vi "Sensors_Scale.vi"() -> ()   [LabVIEW 2017]
uses:
  <vilib>/DAQmx/read.llb/DAQmx Read (Analog 1D Wfm NChan NSamp).vi
  <vilib>/DAQmx/miscellaneous.llb/DAQmx Fill In Error Info.vi
panel:
  out "weight (g)":dbl format="%#_13g"
  out "?":cluster{timestamp[], dbl[]}(graph)={[timestamp(3602780680.000294 s since 1904-01-01), timestamp(3602780680.1853123 s since 1904-01-01), timestamp(3602780680.372331 s since 1904-01-01), timestamp(3602780680.5593495 s since 1904-01-01), timestamp(3602780680.747369 s since 1904-01-01), timestamp(3602780680.9313874 s since 1904-01-01), timestamp(3602780681.120406 s since 1904-01-01), timestamp(3602780681.309425 s since 1904-01-01), timestamp(3602780681.4954433 s since 1904-01-01), timestamp(3602780681.6844625 s since 1904-01-01), timestamp(3602780681.871481 s since 1904-01-01), timestamp(3602780682.0585 s since 1904-01-01), timestamp(3602780682.2445183 s since 1904-01-01), timestamp(3602780682.4305367 s since 1904-01-01), timestamp(3602780682.6185555 s since 1904-01-01), timestamp(3602780682.8075743 s since 1904-01-01), timestamp(3602780682.9955935 s since 1904-01-01), timestamp(3602780683.183612 s since 1904-01-01), timestamp(3602780683.371631 s since 1904-01-01), timestamp(3602780683.56065 s since 1904-01-01), timestamp(3602780683.7476687 s since 1904-01-01), timestamp(3602780683.9326873 s since 1904-01-01), timestamp(3602780684.1167054 s since 1904-01-01), timestamp(3602780684.304724 s since 1904-01-01), timestamp(3602780684.492743 s since 1904-01-01), timestamp(3602780684.680762 s since 1904-01-01), timestamp(3602780684.8677807 s since 1904-01-01), timestamp(3602780685.0578 s since 1904-01-01), timestamp(3602780685.244818 s since 1904-01-01), timestamp(3602780685.432837 s since 1904-01-01)], [0.21837152908225832, 0.21742377911483501, 0.21031033814915645, 0.2086503005079301, 0.21884613322679414, 0.22074219760114033, 0.21125840768619142, 0.21932122763939432, 0.23473182361237477, 0.2444530148877071, 0.20770159564161617, 0.22524839457404866, 0.22667064865852637, 0.20628031893126675, 0.2335451032209548, 0.2169493088130814, 0.23188682444882147, 0.2193204281648633, 0.23781582193533168, 0.2190824597701706, 0.22382541061956118, 0.20746577490400142, 0.21813546462485434, 0.2209789641439528, 0.2205049837107893, 0.2292782030754168, 0.21410368192326956, 0.223114304440994, 0.2330717025481377, 0.23520626745287387]}
  in  "Clear Data":bool
  out "output cluster":T1={"Dynamic Data"=[{"t0"=timestamp(3602781702.123506 s since 1904-01-01), "dt"=0.001, "Y"=[-49.920074642439154, -49.92818457064587, -49.93629449885258, -49.93629449885258, -49.92818457064587, -49.91196471423243, -49.93629449885258, -49.944404427059304, -49.920074642439154, -49.920074642439154, -49.93629449885258, -49.93629449885258, -49.93629449885258, -49.920074642439154, -49.93629449885258, -49.93629449885258, -49.93629449885258, -49.92818457064587, -49.93629449885258, -49.92818457064587, -49.96062428347275, -49.92818457064587, -49.91196471423243, -49.93629449885258, -49.93629449885258, -49.92818457064587, -49.92818457064587, -49.920074642439154, -49.93629449885258, -49.93629449885258, -49.93629449885258, -49.920074642439154, -49.92818457064587, -49.952514355266025, -49.92818457064587, -49.92818457064587, -49.93629449885258, -49.92818457064587, -49.92818457064587, -49.93629449885258, -49.92818457064587, -49.93629449885258, -49.944404427059304, -49.93629449885258, -49.920074642439154, -49.92818457064587, -49.944404427059304, -49.93629449885258, -49.93629449885258, -49.92818457064587, -49.92818457064587, -49.93629449885258, -49.92818457064587, -49.920074642439154, -49.93629449885258, -49.93629449885258, -49.93629449885258, -49.920074642439154, -49.920074642439154, -49.93629449885258, -49.93629449885258, -49.920074642439154, -49.93629449885258, -49.93629449885258, -49.92818457064587, -49.92818457064587, -49.93629449885258, -49.92818457064587, -49.944404427059304, -49.93629449885258, -49.91196471423243, -49.92818457064587, -49.952514355266025, -49.952514355266025, -49.920074642439154, -49.92818457064587, -49.952514355266025, -49.92818457064587, -49.92818457064587, -49.92818457064587, -49.92818457064587, -49.93629449885258, -49.92818457064587, -49.91196471423243, -49.920074642439154, -49.92818457064587, -49.92818457064587, -49.920074642439154, -49.92818457064587, -49.944404427059304, -49.93629449885258, -49.91196471423243, -49.944404427059304, -49.93629449885258, -49.93629449885258, -49.920074642439154, -49.93629449885258, -49.944404427059304, -49.944404427059304, -49.92818457064587], "attributes"=variant("NI_ChannelName"=variant(string "CCP"), "NI_UnitDescription"=variant(string "psi"))}, {"t0"=timestamp(3602781702.12352 s since 1904-01-01), "dt"=0.001, "Y"=[-49.944404427059304, -49.920074642439154, -49.944404427059304, -49.92818457064587, -49.92818457064587, -49.96062428347275, -49.93629449885258, -49.90385478602571, -49.92818457064587, -49.96062428347275, -49.92818457064587, -49.91196471423243, -49.920074642439154, -49.93629449885258, -49.93629449885258, -49.92818457064587, -49.92818457064587, -49.93629449885258, -49.96062428347275, -49.93629449885258, -49.90385478602571, -49.92818457064587, -49.93629449885258, -49.93629449885258, -49.91196471423243, -49.92818457064587, -49.920074642439154, -49.952514355266025, -49.920074642439154, -49.91196471423243, -49.92818457064587, -49.968734211679475, -49.92818457064587, -49.89574485781899, -49.92818457064587, -49.944404427059304, -49.944404427059304, -49.92818457064587, -49.91196471423243, -49.93629449885258, -49.952514355266025, -49.93629449885258, -49.90385478602571, -49.92818457064587, -49.96062428347275, -49.93629449885258, -49.90385478602571, -49.93629449885258, -49.93629449885258, -49.944404427059304, -49.91196471423243, -49.91196471423243, -49.93629449885258, -49.952514355266025, -49.944404427059304, -49.90385478602571, -49.92818457064587, -49.96062428347275, -49.92818457064587, -49.89574485781899, -49.920074642439154, -49.93629449885258, -49.92818457064587, -49.920074642439154, -49.93629449885258, -49.92818457064587, -49.92818457064587, -49.944404427059304, -49.91196471423243, -49.92818457064587, -49.952514355266025, -49.93629449885258, -49.91196471423243, -49.92818457064587, -49.944404427059304, -49.93629449885258, -49.920074642439154, -49.92818457064587, -49.92818457064587, -49.952514355266025, -49.92818457064587, -49.920074642439154, -49.93629449885258, -49.96062428347275, -49.93629449885258, -49.91196471423243, -49.92818457064587, -49.952514355266025, -49.944404427059304, -49.90385478602571, -49.93629449885258, -49.952514355266025, -49.93629449885258, -49.89574485781899, -49.93629449885258, -49.952514355266025, -49.92818457064587, -49.90385478602571, -49.92818457064587, -49.952514355266025], "attributes"=variant("NI_ChannelName"=variant(string "PNP"), "NI_UnitDescription"=variant(string "psi"))}, {"t0"=timestamp(3602781702.123534 s since 1904-01-01), "dt"=0.001, "Y"=[-0.08740270774735379, -0.08738851537299203, -0.08734593824990676, -0.0873601306242685, -0.08738851537299203, -0.08741690012171555, -0.08738851537299203, -0.0873601306242685, -0.08740270774735379, -0.0874310924960773, -0.08737432299863027, -0.08731755350118324, -0.08737432299863027, -0.08738851537299203, -0.08737432299863027, -0.08734593824990676, -0.08737432299863027, -0.08737432299863027, -0.08740270774735379, -0.08738851537299203, -0.08734593824990676, -0.08738851537299203, -0.08741690012171555, -0.08740270774735379, -0.087331745875545, -0.0873601306242685, -0.08737432299863027, -0.08740270774735379, -0.08737432299863027, -0.087331745875545, -0.08737432299863027, -0.08744528487043908, -0.08737432299863027, -0.08731755350118324, -0.08737432299863027, -0.08740270774735379, -0.08738851537299203, -0.08734593824990676, -0.0873601306242685, -0.08738851537299203, -0.08740270774735379, -0.0873601306242685, -0.087331745875545, -0.08737432299863027, -0.08741690012171555, -0.08738851537299203, -0.08731755350118324, -0.08737432299863027, -0.08740270774735379, -0.08738851537299203, -0.0873601306242685, -0.0873601306242685, -0.08738851537299203, -0.08741690012171555, -0.08738851537299203, -0.087331745875545, -0.0873601306242685, -0.0874310924960773, -0.08738851537299203, -0.08731755350118324, -0.08738851537299203, -0.08741690012171555, -0.08738851537299203, -0.087331745875545, -0.08737432299863027, -0.08738851537299203, -0.08738851537299203, -0.08738851537299203, -0.08734593824990676, -0.08737432299863027, -0.0874310924960773, -0.08737432299863027, -0.087331745875545, -0.08740270774735379, -0.0874310924960773, -0.0873601306242685, -0.0873601306242685, -0.08738851537299203, -0.08737432299863027, -0.08740270774735379, -0.08737432299863027, -0.08737432299863027, -0.08740270774735379, -0.0874310924960773, -0.08740270774735379, -0.0873601306242685, -0.08737432299863027, -0.08741690012171555, -0.08737432299863027, -0.087331745875545, -0.08738851537299203, -0.08741690012171555, -0.08737432299863027, -0.087331745875545, -0.08737432299863027, -0.08744528487043908, -0.08737432299863027, -0.08734593824990676, -0.08738851537299203, -0.0874310924960773], "attributes"=variant("NI_ChannelName"=variant(string "Fuel Flow"), "NI_UnitDescription"=variant(string "lpm"))}, {"t0"=timestamp(3602781702.123548 s since 1904-01-01), "dt"=0.001, "Y"=[-7.47842015345857, -7.47842015345857, -7.482799514690198, -7.480609834074384, -7.482799514690198, -7.484989195306012, -7.480609834074384, -7.47842015345857, -7.480609834074384, -7.480609834074384, -7.482799514690198, -7.482799514690198, -7.482799514690198, -7.480609834074384, -7.482799514690198, -7.480609834074384, -7.480609834074384, -7.482799514690198, -7.482799514690198, -7.484989195306012, -7.480609834074384, -7.482799514690198, -7.482799514690198, -7.480609834074384, -7.482799514690198, -7.480609834074384, -7.480609834074384, -7.480609834074384, -7.480609834074384, -7.482799514690198, -7.480609834074384, -7.480609834074384, -7.482799514690198, -7.47842015345857, -7.480609834074384, -7.482799514690198, -7.482799514690198, -7.482799514690198, -7.480609834074384, -7.480609834074384, -7.482799514690198, -7.484989195306012, -7.47842015345857, -7.482799514690198, -7.482799514690198, -7.482799514690198, -7.480609834074384, -7.480609834074384, -7.480609834074384, -7.482799514690198, -7.480609834074384, -7.482799514690198, -7.482799514690198, -7.480609834074384, -7.480609834074384, -7.47842015345857, -7.47842015345857, -7.482799514690198, -7.482799514690198, -7.480609834074384, -7.480609834074384, -7.480609834074384, -7.482799514690198, -7.480609834074384, -7.480609834074384, -7.47842015345857, -7.480609834074384, -7.480609834074384, -7.482799514690198, -7.480609834074384, -7.482799514690198, -7.480609834074384, -7.47842015345857, -7.482799514690198, -7.476230472842756, -7.482799514690198, -7.480609834074384, -7.482799514690198, -7.480609834074384, -7.480609834074384, -7.480609834074384, -7.480609834074384, -7.480609834074384, -7.482799514690198, -7.480609834074384, -7.480609834074384, -7.482799514690198, -7.480609834074384, -7.480609834074384, -7.480609834074384, -7.480609834074384, -7.480609834074384, -7.47842015345857, -7.482799514690198, -7.480609834074384, -7.482799514690198, -7.482799514690198, -7.47842015345857, -7.480609834074384, -7.480609834074384], "attributes"=variant("NI_ChannelName"=variant(string "Water Flow"), "NI_UnitDescription"=variant(string "lpm"))}], "Dynamic Data"=[{"t0"=timestamp(3602781702.223506 s since 1904-01-01), "dt"=0.001, "Y"=[-49.931671839774744], "attributes"=variant("NI_ChannelName"=variant(string "CCP (Arith. Mean)"), "NI_OriginalChannelName"=variant(string "CCP"), "NI_UnitDescription"=variant(string "psi"))}, {"t0"=timestamp(3602781702.2235203 s since 1904-01-01), "dt"=0.001, "Y"=[-49.931185244082364], "attributes"=variant("NI_ChannelName"=variant(string "PNP (Arith. Mean)"), "NI_OriginalChannelName"=variant(string "PNP"), "NI_UnitDescription"=variant(string "psi"))}, {"t0"=timestamp(3602781702.223534 s since 1904-01-01), "dt"=0.001, "Y"=[-0.0873795741771441], "attributes"=variant("NI_ChannelName"=variant(string "Fuel Flow (Arith. Mean)"), "NI_OriginalChannelName"=variant(string "Fuel Flow"), "NI_UnitDescription"=variant(string "lpm"))}, {"t0"=timestamp(3602781702.223548 s since 1904-01-01), "dt"=0.001, "Y"=[-7.481244841452965], "attributes"=variant("NI_ChannelName"=variant(string "Water Flow (Arith. Mean)"), "NI_OriginalChannelName"=variant(string "Water Flow"), "NI_UnitDescription"=variant(string "lpm"))}], "Dynamic Data"=[], "Dynamic Data Type"=[]}
  out "file size TDMS":dbl=132.859375
  in  "Save Data TDMS":bool=TRUE
  out "TDMS file out":refnum<k34>
  out "TDMS error out":errorcluster
  in  "Stop":bool
  in  "Tab Control":enum32{"File", "Setup"}(tab)=enum."Setup"
  in  "base path":path=path "E:/Tests"
  out "file path":path=path "E:/Tests/2018-03-01/Run1_Sensors.tdms"
  in  "Filename":string="Run1_Sensors"
  in  "task/channels in":refnum<k21>="Current_1"
  in  "# HVOF":i32=4
  in  "Minimum time between \nreadings [ms]":u32=100
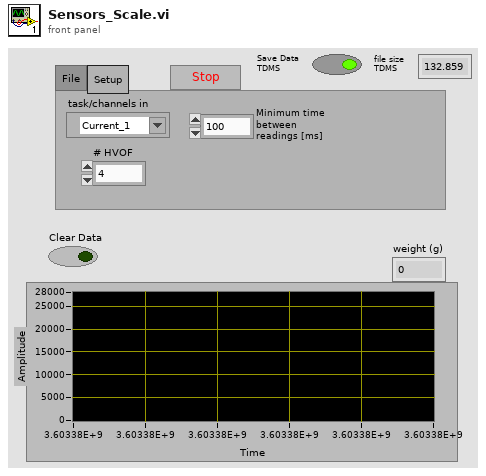
[diagram p1: front panel]
types:
  T1 = cluster{"Dynamic Data":dynamicdata, "Dynamic Data":dynamicdata, "Dynamic Data":dynamicdata, "Dynamic Data Type":dynamicdata}
  T2 = enum16{"open", "open or create", "create or replace", "create", "open (read-only)"}
  T3 = cluster{waveform(dbl)[], "Arithmetic Mean":dynamicdata, waveform(dbl)[], "Arithmetic Mean":dynamicdata}
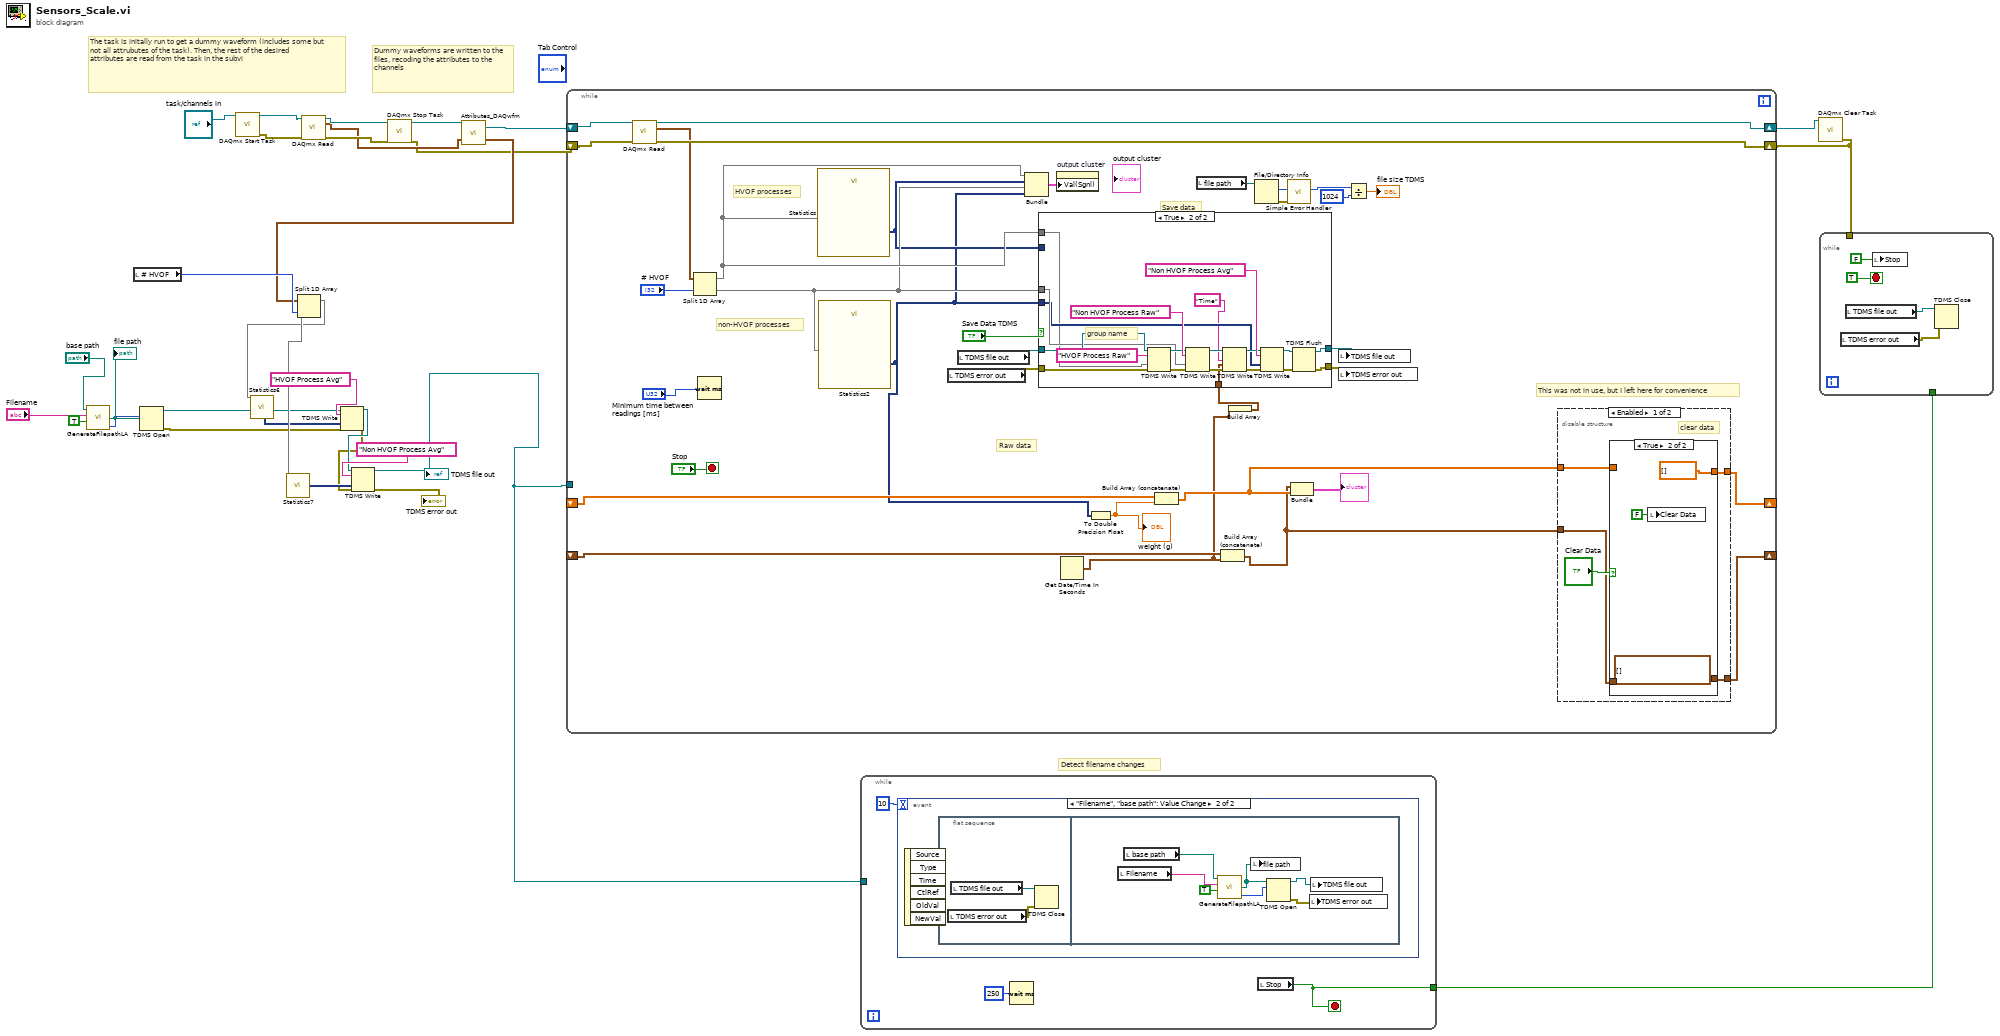
[diagram p0: block diagram]
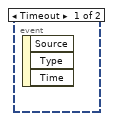
[diagram p5: hidden frame]
diagram:
  # "Detect filename changes"
  # "Dummy waveforms are written to the files, recoding the attributes to the channels"
  # "The task is initally run to get a dummy waveform (includes some but not all attrubutes of the task). Then, the rest of the desired attributes are read from the task in the subvi"
  n1 = call "GenerateFilepathLA.vi"("Auto Date folder"=TRUE, "Filename"="Filename", "base path"="base path") -> ("operation (0:open)"=w13:T2, "file path"=w12:path)  [unwired: 1 in, 1 out]
  "file path" <- w12
  n2 = local read "# HVOF"() -> (w15:i32)
  n3 = TDMS Open(10:w13, 11:w12) -> (0:w6:errorcluster, 3:w7:refnum<k34>)  [unwired: 5 in]
  n4 = call <vilib>:"DAQmx Start Task.vi"("task/channels in"="task/channels in") -> ("task out"=w29:refnum<k21>, "error out"=w28:errorcluster)  [unwired: 13 in]
  n5 = call-poly <vilib>:"DAQmx Read.vi"("task/channels in"=w29, "error in"=w28) -> ("task out"=w27:refnum<k21>, "data"=w24:waveform(dbl)[], "error out"=w26:errorcluster)  [unwired: 11 in]
  n6 = call <vilib>:"DAQmx Stop Task.vi"("task/channels in"=w27, "error in"=w26) -> ("task out"=w25:refnum<k21>, "error out"=w1:errorcluster)  [unwired: 12 in]
  n7 = call "Attributes_DAQwfm.vi"("data"=w24, "Refnum in"=w25) -> ("Array"=w8:waveform(dbl)[], "Refnum in 2"=w23:refnum<k21>)
  n8 = Split 1D Array(array=w8, index=w15) -> (first subarray=w18:waveform(dbl)[], second subarray=w20:waveform(dbl)[])
  n9 = call "Statistics6"("Signals"=w18) -> ("Arithmetic Mean"=w19:dynamicdata)  [unwired: 24 in, 2 out]
  n10 = call "Statistics7"("Signals"=w20) -> ("Arithmetic Mean"=w21:dynamicdata)  [unwired: 24 in, 2 out]
  n11 = TDMS Write(0:w7, 5:"HVOF Process Avg" ("group name in (Untitled)"), 9:w19, 11:w6) -> (4:w5:refnum<k34>, 15:w4:errorcluster)  [unwired: 2 in, 2 out]
  n12 = TDMS Write(0:w5, 5:"Non HVOF Process Avg" ("group name in (Untitled)"), 9:w21, 11:w4) -> (4:w3:refnum<k34>, 15:→"TDMS error out":errorcluster)  [unwired: 2 in, 2 out]
  "TDMS file out" <- w3
  n13 = while {
    shift-right: [w64] -> w31
    shift-left: w1 -> [w60]
    tunnel: w3 -> [_]
    shift-right: [w61] -> w22
    shift-left: w23 -> [w62]
    shift-right: [w36] -> _
    shift-left: _ -> [w42]
    shift-right: [w34] -> _
    shift-left: _ -> [w41]
    stop <- "Stop" stop-if-true
    # "This was not in use, but I left here for convenience"
    # "Save data"
    # "non-HVOF processes"
    # "HVOF processes"
    # "Raw data"
    n14 = call-poly <vilib>:"DAQmx Read.vi"("task/channels in"=w62, "error in"=w60) -> ("task out"=w61:refnum<k21>, "data"=w58:waveform(dbl)[], "error out"=w64:errorcluster)  [unwired: 11 in]
    n15 = Split 1D Array(array=w58, index="# HVOF") -> (first subarray=w56:waveform(dbl)[], second subarray=w45:waveform(dbl)[])
    n16 = Wait (ms)(milliseconds to wait="Minimum time between \nreadings [ms]") -> ()  [unwired: 1 out]
    n17 = call "Statistics"("Signals"=w56) -> ("Arithmetic Mean"=w43:dynamicdata)  [unwired: 24 in, 2 out]
    n18 = call "Statistics2"("Signals"=w45) -> ("Arithmetic Mean"=w39:dynamicdata)  [unwired: 24 in, 2 out]
    n19 = local read "TDMS error out"() -> (w51:errorcluster)
    n20 = local read "TDMS file out"() -> (w50:refnum<k34>)
    n21 = Bundle(w56, "Arithmetic Mean"=w43, w45, "Arithmetic Mean"=w39) -> (w44:T3)  [unwired: 1 in]
    n22 = property on="output cluster" class="Clust (strict)"("Val(Sgnl)"=w44) -> ()  [unwired: 2 in, 2 out]
    n23 = Get Date/Time In Seconds() -> (seconds since 1Jan1904=w33:timestamp)
    n24 = To Double Precision Float(number=w39) -> (double precision float=w38:dbl)
    "weight (g)" <- w38
    n25 = Build Array (concatenate)(w42, w38) -> (w37:dbl[])
    n26 = local read "file path"() -> (w53:path)
    n27 = Build Array (concatenate)(w41, w33) -> (w35:timestamp[])
    n28 = Build Array(w33) -> (w32:timestamp[])
    n29 = case shown="True" "Save Data TDMS" {
      tunnel: w50 -> [w76 w91]
      tunnel: w51 -> [w75 w87]
      tunnel: [w76 w96] -> w47
      tunnel: [w75 w95] -> w46
      tunnel: w43 -> [_ _]
      tunnel: w45 -> [_ w81]
      tunnel: w39 -> [_ w80]
      tunnel: w56 -> [_ w79]
      tunnel: w32 -> [_ w78]
      frame False {
      }
      frame True {
        # "group name"
        n30 = TDMS Write(0:w91, 5:"HVOF Process Raw" ("group name in (Untitled)"), 9:w79, 11:w87) -> (4:w90:refnum<k34>, 15:w86:errorcluster)  [unwired: 2 in, 2 out]
        n31 = TDMS Write(0:w90, 5:"Non HVOF Process Raw" ("group name in (Untitled)"), 9:w81, 11:w86) -> (4:w89:refnum<k34>, 15:w85:errorcluster)  [unwired: 2 in, 2 out]
        n32 = TDMS Write(0:w89, 7:"Time", 9:w78, 11:w85) -> (4:w88:refnum<k34>, 15:w84:errorcluster)  [unwired: 2 in, 2 out]
        n33 = TDMS Write(0:w88, 5:"Non HVOF Process Avg" ("group name in (Untitled)"), 9:w80, 11:w84) -> (4:w83:refnum<k34>, 15:w82:errorcluster)  [unwired: 2 in, 2 out]
        n34 = TDMS Flush(4:w82, 7:w83) -> (0:w95:errorcluster, 3:w96:refnum<k34>)
      }
    }
    n35 = File/Directory Info(path=w53) -> (size=w55:i64, error out=w52:errorcluster)  [unwired: 1 in, 5 out]
    n36 = call <vilib>:"Simple Error Handler.vi"("error in (no error)"=w52) -> ()  [unwired: 1 in, 8 out]
    n37 = Bundle(w35, w37) -> (→"?":cluster{timestamp[], dbl[]})  [unwired: 1 in]
    n38 = local write "TDMS file out"(w47) -> ()
    n39 = local write "TDMS error out"(w46) -> ()
    n40 = Divide(x=w55, y=i64 1024) -> (x/y=→"file size TDMS":dbl)
    n41 = disable-structure shown="Enabled" {
      disable-tunnel: w37 -> [w68 _]
      disable-tunnel: [w67 _] -> w36
      disable-tunnel: [w66 _] -> w34
      disable-tunnel: w35 -> [w65 _]
      frame Enabled {
        # "clear data"
        n42 = case shown="True" "Clear Data" {
          tunnel: w68 -> [w71 _]
          tunnel: [w71 dbl[] []] -> w67
          tunnel: [w70 timestamp[] []] -> w66
          tunnel: w65 -> [w70 _]
          frame False {
          }
          frame True {
            n43 = local write "Clear Data"(FALSE ("Clear Data")) -> ()
          }
        }
      }
      frame Disabled {
      }
    }
  }
  n44 = while {
    tunnel: w3 -> [_]
    tunnel: [w97] -> w2
    stop <- w97 stop-if-true
    n45 = event shown="[1] \"Filename\", \"base path\": Value Change" {
      selector: _ -> [_ _]
      dyn-events: _ -> [_ _]
      timeout: 10 -> [_ _]
      event Timeout {
        n46 = event-data() -> ()  [unwired: 1 in, 3 out]
      }
      event "Filename", "base path": Value Change {
        n47 = event-data() -> ()  [unwired: 1 in, 6 out]
        n48 = flat-sequence {
          frame #0 {
            n49 = local read "TDMS error out"() -> (w101:errorcluster)
            n50 = local read "TDMS file out"() -> (w100:refnum<k34>)
            n51 = TDMS Close(8:w101, 11:w100) -> ()  [unwired: 2 out]
          }
          frame #1 {
            n52 = local read "Filename"() -> (w108:string)
            n53 = local read "base path"() -> (w107:path)
            n54 = call "GenerateFilepathLA.vi"("Auto Date folder"=TRUE, "Filename"=w108, "base path"=w107) -> ("operation (0:open)"=w104:T2, "file path"=w106:path)  [unwired: 1 in, 1 out]
            n55 = local write "file path"(w106) -> ()
            n56 = TDMS Open(10:w104, 11:w106) -> (0:w102:errorcluster, 3:w103:refnum<k34>)  [unwired: 5 in]
            n57 = local write "TDMS error out"(w102) -> ()
            n58 = local write "TDMS file out"(w103) -> ()
          }
        }
      }
    }
    n59 = Wait (ms)(milliseconds to wait=u32 250) -> ()  [unwired: 1 out]
    n60 = local read "Stop"() -> (w97:bool)
  }
  n61 = call <vilib>:"DAQmx Clear Task.vi"("task in"=w22, "error in"=w31) -> ()  [unwired: 13 in, 1 out]
  n62 = while {
    tunnel: w31 -> [_]
    tunnel: w2 -> [_]
    stop <- TRUE stop-if-true
    n63 = local read "TDMS error out"() -> (w110:errorcluster)
    n64 = local read "TDMS file out"() -> (w109:refnum<k34>)
    n65 = local write "Stop"(FALSE ("stop_vi")) -> ()
    n66 = TDMS Close(8:w110, 11:w109) -> ()  [unwired: 2 out]
  }
